vi "Handle Notification.vi"(8 "error in (no error)":errorcluster, 9 "Payload":string, 10 "Notification Type":string, 11 "Test Sequencer in":refnum<class "Sequencer with Output Values.lvclass">) -> (0 "error out":errorcluster, 3 "Test Sequencer out":refnum<class "Sequencer with Output Values.lvclass">)   [LabVIEW 2020, in "Sequencer with Output Values.lvlib" / "Sequencer with Output Values.lvclass"]
uses:
  Sequencer with Output Values.lvclass
  Sequencer with Output Values.lvclass/Sequencer with Output Values.ctl
  Global Strings.vi
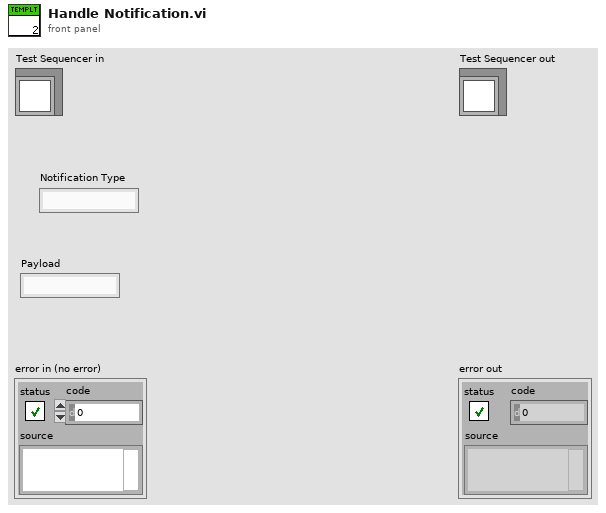
[diagram p1: front panel]
types:
  T1 = typedef "Sequencer with Output Values.lvlib/Sequencer with Output Values.lvclass/Params.ctl" = cluster{"Step Values":T2[], "Only Execute When Test Running":bool, "Reset Sequence When Test Starts":bool, "Current Sequence ID":u32, "Total Iterations":u32, "Current Step Start Timestamp":dbl, "Number of Sequence Steps":i32, "Num of Analog Channels":i32, "Num of Digital Channels":i32, "Delay Before Starting Sequence":dbl, "Show UI":bool, "Time Remaining":dbl, "Test Running":bool, "Pause Timestamp":dbl, "Default Analog Values":dbl[], "Default Digital Values":bool[]}
  T2 = typedef "Sequencer with Output Values.lvlib/Sequencer with Output Values.lvclass/Step Settings.ctl" = cluster{"Duration":dbl, "Mode":string, "Delay Between Values":dbl, "Analog Values":string[], "Digital Values":string[]}
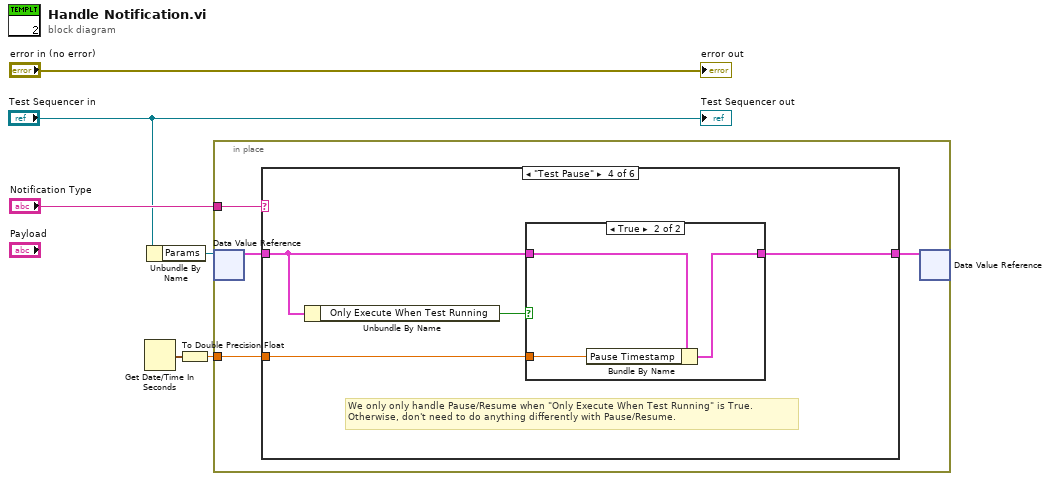
[diagram p0: block diagram]
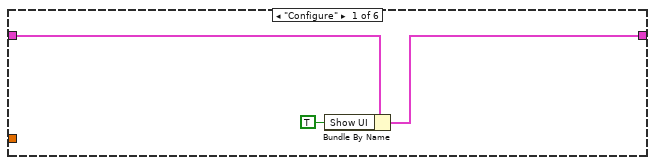
[diagram p2: hidden frame]
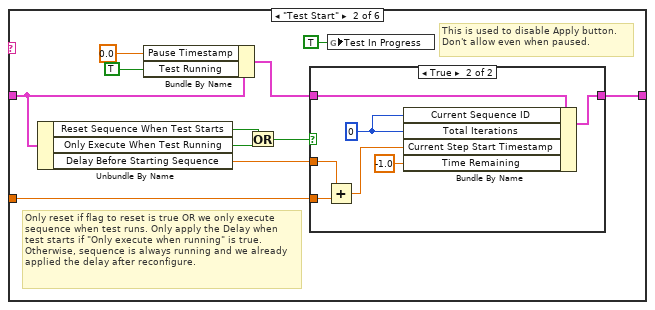
[diagram p3: hidden frame]
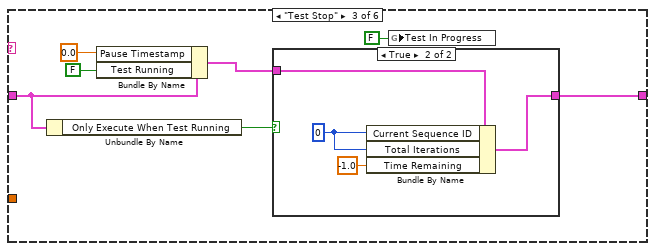
[diagram p5: hidden frame]
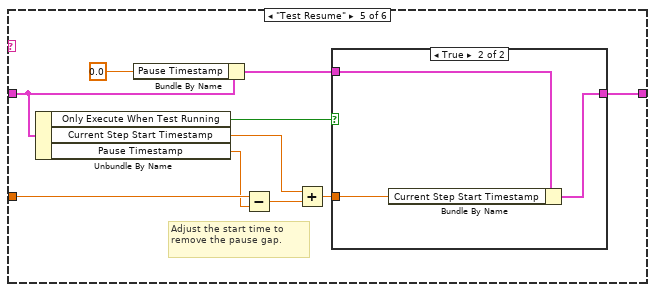
[diagram p8: hidden frame]
diagram:
  n1 = Get Date/Time In Seconds() -> (seconds since 1Jan1904=w2:timestamp)
  n2 = Unbundle By Name("Test Sequencer in") -> ("Params"=w3:refnum<data-value>)
  n3 = To Double Precision Float(number=w2) -> (double precision float=w1:dbl)
  n4 = in-place {
    in-place-border: "Notification Type" -> [w10]
    in-place-border: w1 -> [w7]
    n5 = in-place-dvr #1(w3) -> (w9:T1)  [unwired: 1 out]
    n6 = case shown="\"Test Pause\"" w10 {
      tunnel: w9 -> [w12 w20 w38 w46 w62 w67]
      tunnel: [w11 w19 w35 w48 w56 w67] -> w8
      tunnel: w7 -> [_ w18 _ w47 w61 _]
      frame "Configure" {
        n7 = Bundle By Name(cluster=w12, "Show UI"=TRUE) -> (w11:T1)
      }
      frame "Test Start" {
        # "This is used to disable Apply button. Don't allow even when paused."
        # "Only reset if flag to reset is true OR we only execute sequence when test runs. Only apply the Delay when test starts if \"Only execute when running\" is true. Otherwise, sequence is always running and we already applied the delay after reconfigure."
        n8 = Unbundle By Name(w20) -> ("Reset Sequence When Test Starts"=w22:bool, "Only Execute When Test Running"=w15:bool, "Delay Before Starting Sequence"=w14:dbl)
        n9 = Bundle By Name(cluster=w20, "Pause Timestamp"=0.0, "Test Running"=TRUE) -> (w23:T1)
        n10 = Or(x=w22, y=w15) -> (x .or. y?=w21:bool)
        n11 = case shown="True" w21 {
          tunnel: [w25 w32] -> w19
          tunnel: w23 -> [w25 w30]
          tunnel: w18 -> [_ w29]
          tunnel: w14 -> [_ w28]
          frame False {
          }
          frame True {
            w31 = u32 0 ("Total Iterations")
            n12 = Add(x=w28, y=w29) -> (x+y=w27:dbl)
            n13 = Bundle By Name(cluster=w30, "Current Sequence ID"=w31, "Total Iterations"=w31, "Current Step Start Timestamp"=w27, "Time Remaining"=-1.0) -> (w32:T1)
          }
        }
        n14 = global write "Global Strings.vi" "Test In Progress"(TRUE ("Test In Progress")) -> ()
      }
      frame "Test Stop" {
        n15 = Unbundle By Name(w38) -> ("Only Execute When Test Running"=w37:bool)
        n16 = Bundle By Name(cluster=w38, "Pause Timestamp"=0.0, "Test Running"=FALSE) -> (w36:T1)
        n17 = case shown="True" w37 {
          tunnel: w36 -> [w40 w44]
          tunnel: [w40 w42] -> w35
          frame False {
          }
          frame True {
            w43 = u32 0 ("Current Sequence ID")
            n18 = Bundle By Name(cluster=w44, "Current Sequence ID"=w43, "Total Iterations"=w43, "Time Remaining"=-1.0) -> (w42:T1)
          }
        }
        n19 = global write "Global Strings.vi" "Test In Progress"(FALSE ("Test In Progress")) -> ()
      }
      frame "Test Pause" {
        # "We only only handle Pause/Resume when \"Only Execute When Test Running\" is True.\nOtherwise, don't need to do anything differently with Pause/Resume."
        n20 = Unbundle By Name(w46) -> ("Only Execute When Test Running"=w45:bool)
        n21 = case shown="True" w45 {
          tunnel: [w49 w52] -> w48
          tunnel: w47 -> [_ w51]
          tunnel: w46 -> [w49 w50]
          frame False {
          }
          frame True {
            n22 = Bundle By Name(cluster=w50, "Pause Timestamp"=w51) -> (w52:T1)
          }
        }
      }
      frame "Test Resume" {
        # "Adjust the start time to remove the pause gap."
        n23 = Unbundle By Name(w62) -> ("Only Execute When Test Running"=w54:bool, "Current Step Start Timestamp"=w59:dbl, "Pause Timestamp"=w60:dbl)
        n24 = Bundle By Name(cluster=w62, "Pause Timestamp"=0.0) -> (w58:T1)
        n25 = Subtract(x=w61, y=w60) -> (x-y=w55:dbl)
        n26 = Add(x=w59, y=w55) -> (x+y=w57:dbl)
        n27 = case shown="True" w54 {
          tunnel: w58 -> [w63 w66]
          tunnel: w57 -> [_ w65]
          tunnel: [w63 w64] -> w56
          frame False {
          }
          frame True {
            n28 = Bundle By Name(cluster=w66, "Current Step Start Timestamp"=w65) -> (w64:T1)
          }
        }
      }
      frame Default {
      }
    }
    n29 = in-place-dvr #1(w8) -> ()  [unwired: 2 out]
  }
  "error out" <- "error in (no error)"
  "Test Sequencer out" <- "Test Sequencer in"
